vi "Real 32 Converter.vi"(7 "Byte Order (Normal)":T1(ring), 8 "error in (no error)":errorcluster, 10 "Data In":string) -> (0 "error out":errorcluster, 2 "Data Array Out":sgl[](array[numeric]))   [LabVIEW 2018, in "Keithley 3706.lvlib"]
uses:
  <instrlib>/Keithley 3706/Keithley 3706.lvlib
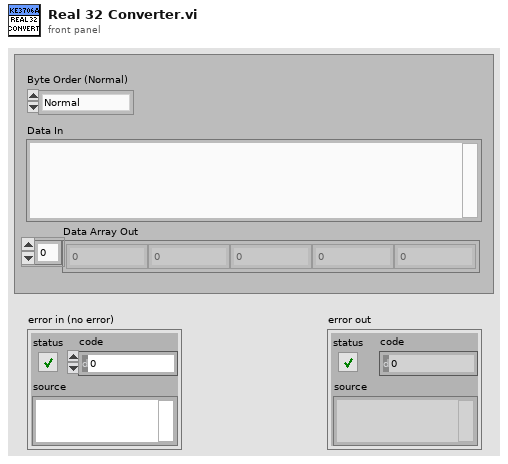
[diagram p1: front panel]
types:
  T1 = enum32{"Normal", "Big Endian", "Little Endian", "Network", "Swapped"}
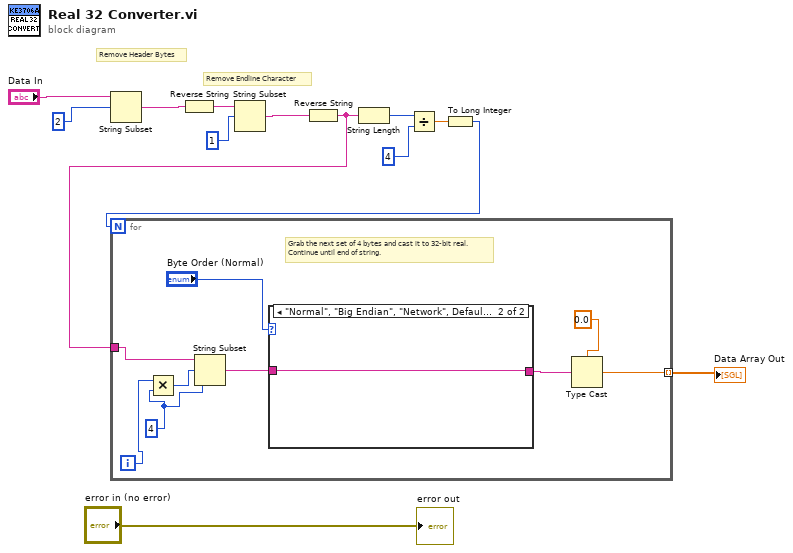
[diagram p0: block diagram]
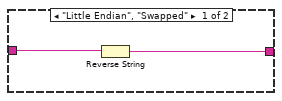
[diagram p2: hidden frame]
diagram:
  # "Remove Endline Character"
  # "Remove Header Bytes"
  n1 = String Subset(string="Data In", offset (0)=2) -> (substring=w10:string)  [unwired: 1 in]
  n2 = Reverse String(1:w10) -> (0:w9:string)
  n3 = String Subset(string=w9, offset (0)=1) -> (substring=w7:string)  [unwired: 1 in]
  n4 = Reverse String(1:w7) -> (0:w2:string)
  n5 = String Length(string=w2) -> (length=w6:i32)
  n6 = Divide(x=w6, y=4) -> (x/y=w4:dbl)
  n7 = To Long Integer(number=w4) -> (32bit integer=w3:i32)
  n8 = for {
    N: w3 -> [_]
    tunnel: w2 -> [w19]
    tunnel: [w14] -> w1 mode=indexing
    i -> [w22]
    w20 = 4
    # "Grab the next set of 4 bytes and cast it to 32-bit real.\nContinue until end of string."
    n9 = Multiply(x=w22, y=w20) -> (x*y=w21:i32)
    n10 = String Subset(string=w19, offset (0)=w21, length (rest)=w20) -> (substring=w17:string)
    n11 = case shown="\"Normal\", \"Big Endian\", \"Network\", Default" "Byte Order (Normal)" {
      tunnel: w17 -> [w24 w25]
      tunnel: [w23 w25] -> w16
      frame "Little Endian", "Swapped" {
        n12 = Reverse String(1:w24) -> (0:w23:string)
      }
      frame "Normal", "Big Endian", "Network", Default {
      }
    }
    n13 = Type Cast(type=sgl 0.0, x=w16) -> (*(type *) &x=w14:sgl)
  }
  "Data Array Out" <- w1
  "error out" <- "error in (no error)"
